vi "Image To Tensor.vi"(8 "error in (no error)":errorcluster, 11 "image data":T1) -> (0 "error out":errorcluster, 2 "Data":sgl[](array[numeric]), 3 "image":picture)   [LabVIEW 2017]
uses:
  <vilib>/picture/picture.llb/imagedata.ctl
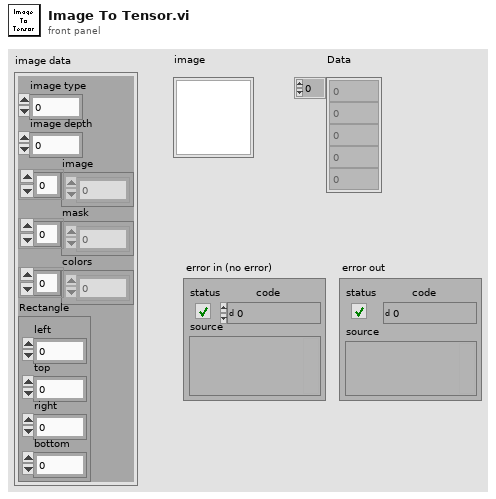
[diagram p1: front panel]
types:
  T1 = typedef "imagedata.ctl" = cluster{"image type":i32, "image depth":i32, "image":u8[], "mask":u8[], "colors":u32[], "Rectangle":cluster{"left":i16, "top":i16, "right":i16, "bottom":i16}}
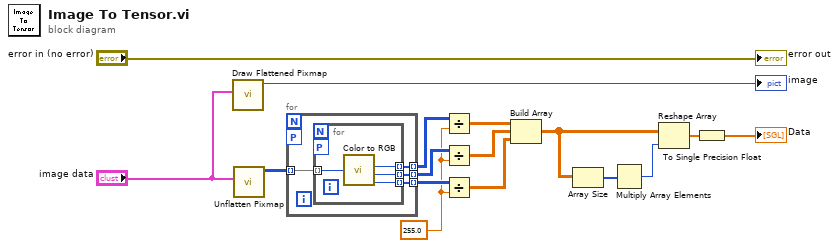
[diagram p0: block diagram]
diagram:
  w4 = 255.0 ("y")
  n1 = call <vilib>:"Draw Flattened Pixmap.vi"("image data"="image data") -> ("new picture"=→"image":picture)  [unwired: 8 in]
  n2 = call <vilib>:"Unflatten Pixmap.vi"("image data"="image data") -> ("24-bit pixmap"=w15:u32[][])  [unwired: 10 out]
  n3 = for {
    tunnel: w15 -> [w20] mode=indexing
    tunnel: [w19] -> w5 mode=indexing
    tunnel: [w18] -> w6 mode=indexing
    tunnel: [w17] -> w7 mode=indexing
    workers-P: _ -> [_]
    n4 = for {
      tunnel: w20 -> [w21] mode=indexing
      tunnel: [w24] -> w19 mode=indexing
      tunnel: [w23] -> w18 mode=indexing
      tunnel: [w22] -> w17 mode=indexing
      workers-P: _ -> [_]
      n5 = call <vilib>:"Color to RGB.vi"("Color"=w21) -> ("R"=w24:u8, "G"=w23:u8, "B"=w22:u8)  [unwired: 1 out]
    }
  }
  n6 = Divide(x=w5, y=w4) -> (x/y=w8:dbl[][])
  n7 = Divide(x=w6, y=w4) -> (x/y=w9:dbl[][])
  n8 = Divide(x=w7, y=w4) -> (x/y=w10:dbl[][])
  n9 = Build Array(w8, w9, w10) -> (w12:dbl[][][])
  n10 = Array Size(array=w12) -> (size(s)=w11:i32[])
  n11 = Multiply Array Elements(1:w11) -> (0:w13:i32)
  n12 = Reshape Array(w12, w13) -> (w14:dbl[])
  n13 = To Single Precision Float(number=w14) -> (single precision float=→"Data":sgl[])
  "error out" <- "error in (no error)"
